vi "lia_fpga.vi"() -> ()   [LabVIEW 2009]
uses:
  <vilib>/eio/EIONode/EIONode.xnode
  <vilib>/rvi/eio/nirviEIOImplementation/nirviEIOImplementation.xnode
  <vilib>/rvi/eio/common/nirviEmuTemplateMethod_noerrors.vi
  <vilib>/rvi/eio/common/nirviEmuClasses.ctl
panel:
  in  "control":i16
  in  "decimation":i16
  in  "stages":i16
  in  "dec":i16
  in  "dec2":i16
  in  "dec1":i16
  out "Accumulator Value":u32
  in  "Signal Amplitude":u16
  in  "Phase Shift":u32
  in  "Accumulator Increment":u32
  in  "Reset Accumulator":bool
  in  "?":bool
  out "Actual Gen Rate (ticks)":u32
  in  "Update Rate (ticks)":u32
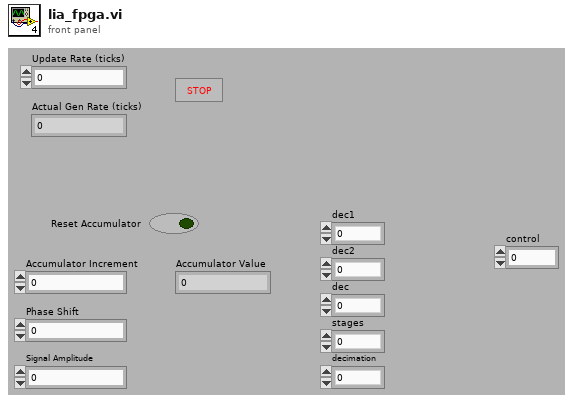
[diagram p1: front panel]
types:
  T1 = typedef "nirviEmuClasses.ctl" = enum16{"IO Read", "IO Write", "Method", "Property Read", "Property Write"}
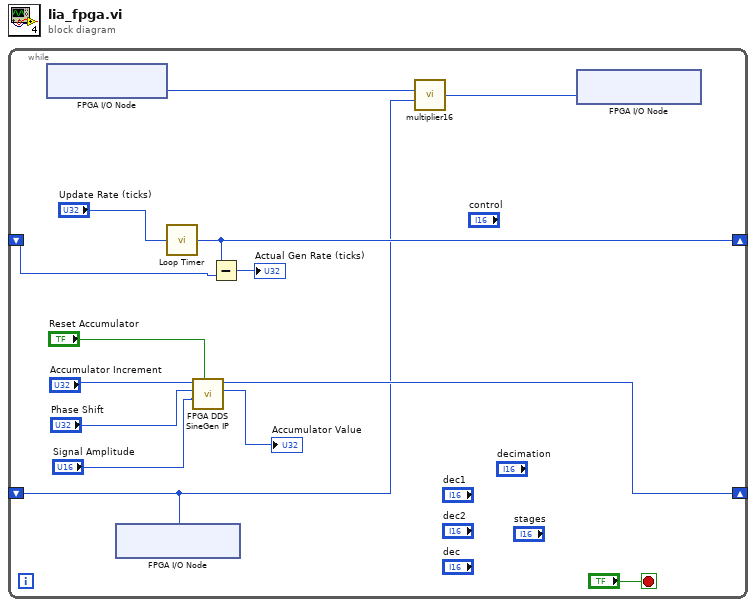
[diagram p0: block diagram]
diagram:
  n1 = while {
    shift-right: [w11] -> _
    shift-left: _ -> [w12]
    shift-right: [w6] -> _
    shift-left: _ -> [w2]
    stop <- "?" stop-if-true
    n2 = xnode "FPGA I/O Node"() -> ("Connector0/AI0"=w3:i16)  [unwired: 1 in, 1 out]
    n3 = xnode "FPGA I/O Node"("Connector0/AO0"=w2) -> ()  [unwired: 1 in, 1 out]
    n4 = call "Loop Timer"("Count(Ticks)"="Update Rate (ticks)") -> ("Tick Count(Ticks)"=w11:u32)
    n5 = call "FPGA DDS SineGen IP.vi"("Reset Accumulator"="Reset Accumulator", "Signal Amplitude (x 2^15)"="Signal Amplitude", "Phase Shift"="Phase Shift", "Accumulator Increment"="Accumulator Increment") -> ("Accumulator Value"=→"Accumulator Value":u32, "Signal Value"=w6:i16)  [unwired: 6 in]
    n6 = Subtract(x=w11, y=w12) -> (x-y=→"Actual Gen Rate (ticks)":u32)
    n7 = call "multiplier16.vi"("Y"=w2, "X"=w3) -> ("XY"=w1:i16)
    n8 = xnode "FPGA I/O Node"("Connector0/AO1"=w1) -> ()  [unwired: 1 in, 1 out]
  }
